vi "Write To Instrument.vi"(8 "error in (no error)":errorcluster, 10 "Write String":string, 11 "VISA resource name":refnum<visa-resource-name>) -> (0 "error out":errorcluster, 3 "VISA resource name out":refnum<visa-resource-name>)   [LabVIEW 2020, in "Temptronic TP04300.lvlib"]
doc: "This VI writes commands and queries to the instrument."
uses:
  Temptronic TP04300.lvlib
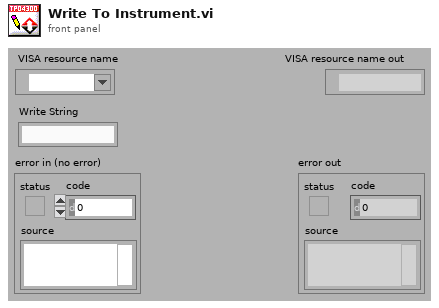
[diagram p1: front panel]
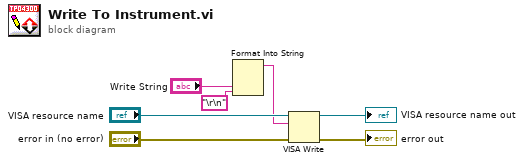
[diagram p0: block diagram]
diagram:
  n1 = Format Into String("Write String", "\r\n") -> (resulting string=w2:string)  [unwired: 3 in, 1 out]
  n2 = VISA Write(VISA resource name="VISA resource name", write buffer=w2, error in (no error)="error in (no error)") -> (VISA resource name out=→"VISA resource name out":refnum<visa-resource-name>, error out=→"error out":errorcluster)  [unwired: 1 out]
